vi "SimpleMotorFF_Calculate.vi"(9 "Accel":dbl, 10 "Vel Sp":dbl, 11 "SIMPLE_MOTOR_FF":T1 {"KnInv" format="%13.4f"; "Ka" format="%13.4f"; "Kv" format="%13.4f"; "Ks" format="%13.4f"}) -> (3 "FeedForward":dbl)   [LabVIEW 2019, in "Trajectory_Library.lvlib"]
doc: "Calculates the feedforward from the gains and setpoints.\n \nParameters:\n - SimpleMotorFF -- Data structure containing constants\n - velocity Setpiont -- The velocity setpoint.\n - acceleration -- The setpoint acceleration. (Note that this could also be calculated\n from desired velocity, previous desired velocity (or actual velocity), and cycle time.) \n \nReturns:\n - FeedForward - The computed feedforward."
uses:
  Trajectory_Library.lvlib
  TypeDef/SIMPLE_MOTOR_FF.ctl
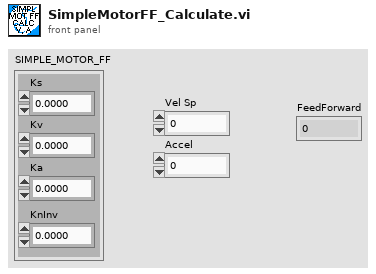
[diagram p1: front panel]
types:
  T1 = typedef "Trajectory_Library.lvlib/SIMPLE_MOTOR_FF.ctl" = cluster{"Ks":dbl, "Kv":dbl, "Ka":dbl, "KnInv":dbl}
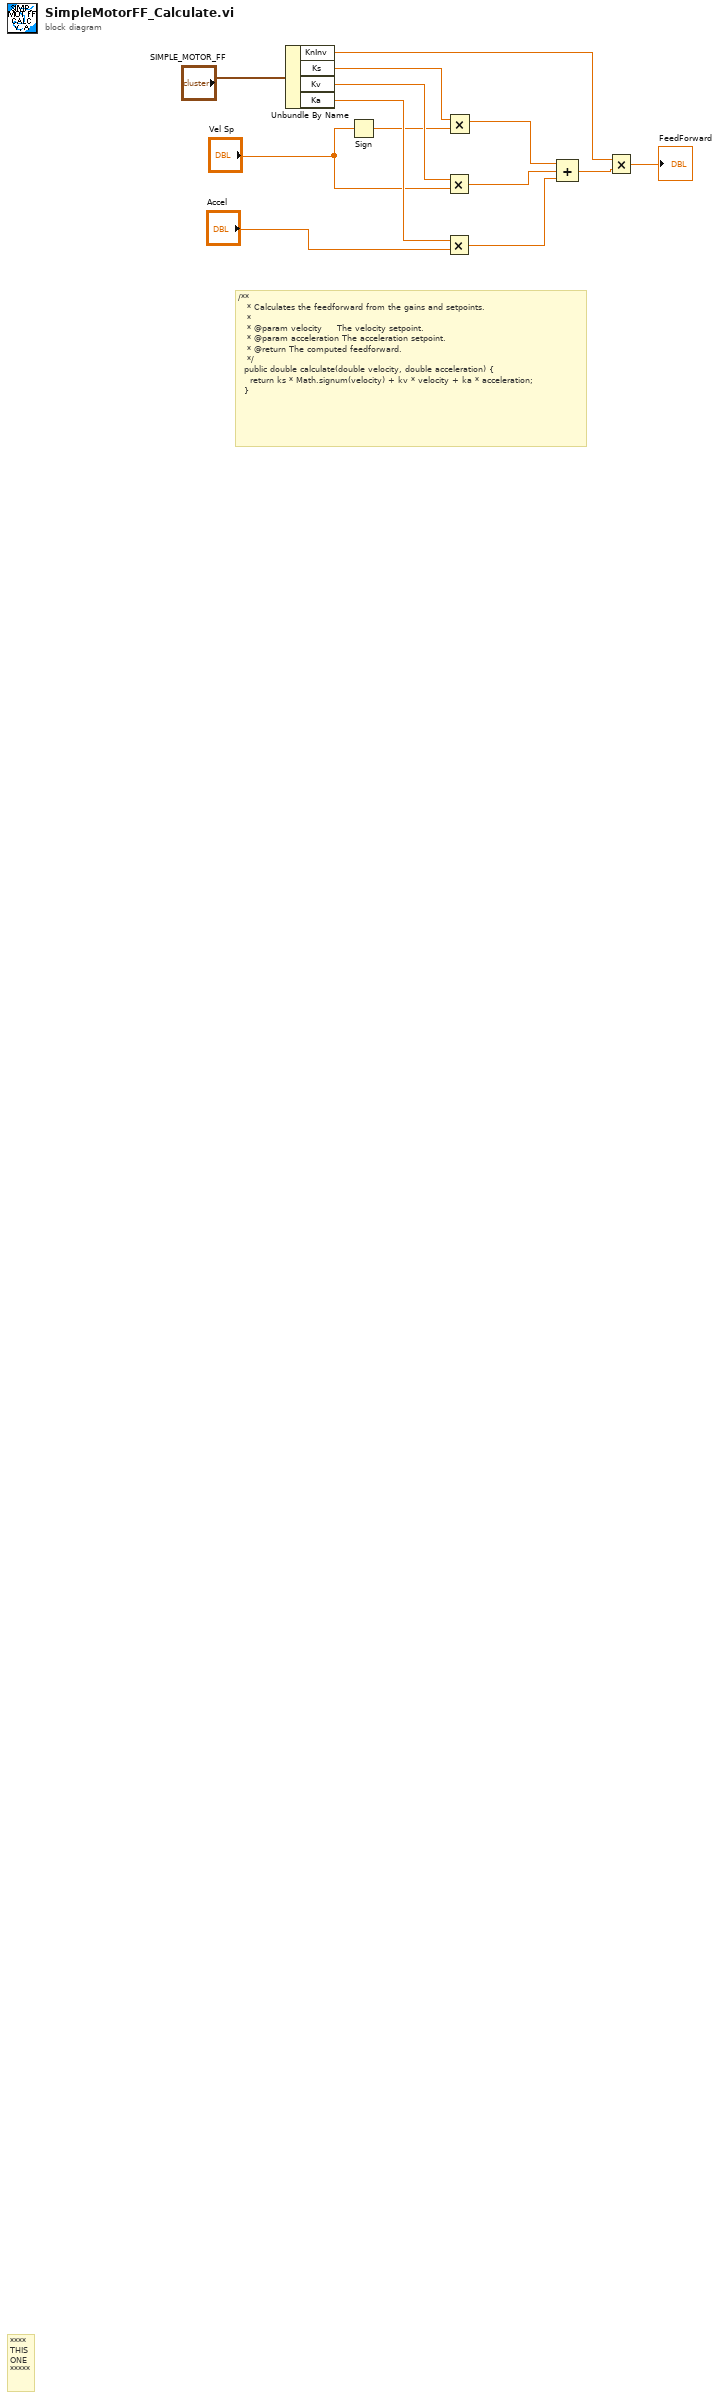
[diagram p0: block diagram]
diagram:
  # "/**\n   * Calculates the feedforward from the gains and setpoints.\n   *\n   * @param velocity     The velocity setpoint.\n   * @param acceleration The acceleration setpoint.\n   * @return The computed feedforward.\n   */\n  public double calculate(double velocity, double acceleration) {\n    return ks * Math.signum(velocity) + kv * velocity + ka * acceleration;\n  }"
  # "****\nTHIS\nONE\n*****"
  n1 = Unbundle By Name("SIMPLE_MOTOR_FF") -> ("KnInv"=w1:dbl, "Ks"=w12:dbl, "Kv"=w11:dbl, "Ka"=w10:dbl)
  n2 = Sign(1:"Vel Sp") -> (0:w8:dbl)
  n3 = Multiply(x=w11, y="Vel Sp") -> (x*y=w5:dbl)
  n4 = Multiply(x=w10, y="Accel") -> (x*y=w4:dbl)
  n5 = Multiply(x=w12, y=w8) -> (x*y=w6:dbl)
  n6 = Compound Arithmetic op=ADD(w6, w5, w4) -> (w3:dbl)
  n7 = Multiply(x=w1, y=w3) -> (x*y=→"FeedForward":dbl)
